vi "FPGA Pulse.vi"(8 "error in (no error)":errorcluster, 11 "fpgaCommand":u8) -> (0 "error out":errorcluster, 3 "function return":i32)   [LabVIEW 2012]
uses:
  x64/Stats.lvlib
  x86/Stats32.lvlib
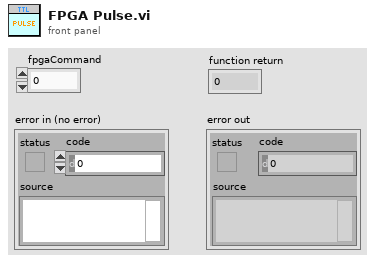
[diagram p1: front panel]
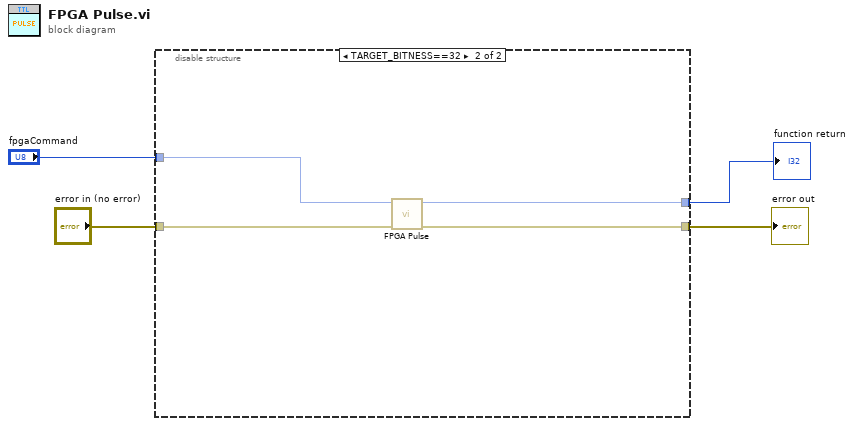
[diagram p0: block diagram]
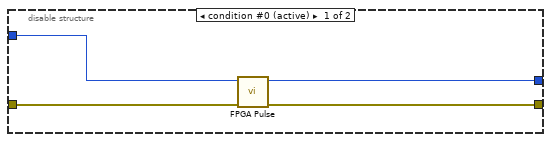
[diagram p2: hidden frame]
diagram:
  n1 = disable-structure shown="TARGET_BITNESS==32" {
    disable-tunnel: "error in (no error)" -> [w8 w10]
    disable-tunnel: [w7 w12] -> w3
    disable-tunnel: [w6 w11] -> w2
    disable-tunnel: "fpgaCommand" -> [w5 w9]
    frame condition #0 (active) {
      n2 = call "FPGA Pulse.vi"("error in (no error)"=w8, "fpgaCommand"=w5) -> ("error out"=w7:errorcluster, "function return"=w6:i32)  [unwired: 8 in]
    }
    frame condition #1 {
      n3 = call "FPGA Pulse.vi"("error in (no error)"=w10, "fpgaCommand"=w9) -> ("error out"=w12:errorcluster, "function return"=w11:i32)  [unwired: 8 in]
    }
  }
  "error out" <- w3
  "function return" <- w2
